vi "Pop Up Button Animator.vi"(5 "Button Ref":refnum<vi>, 7 "Msg Settings":T1={"Grow Time"=0.3, "Msg Time"=0.5, "Shrink Time"=0.1, "Msg Pos"={"Left"=170, "Top"=300}, "Button Size"={"Width"=169, "Height"=93}}, 8 "error in (no error)":errorcluster) -> (0 "error out":errorcluster)   [LabVIEW 2013]
uses:
  Message States.ctl
  <vilib>/Utility/miscctls.llb/LVBoundsTypeDef.ctl
panel:
  out "Message":string
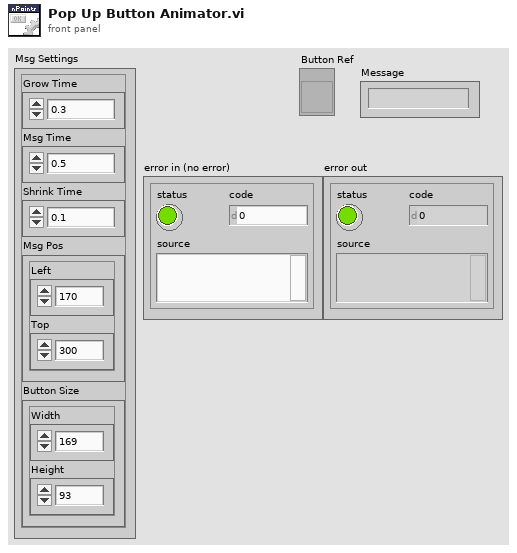
[diagram p1: front panel]
types:
  T1 = cluster{"Grow Time":dbl, "Msg Time":dbl, "Shrink Time":dbl, "Msg Pos":cluster{"Left":i32, "Top":i32}, "Button Size":cluster{"Width":i32, "Height":i32}}
  T2 = typedef "Message States.ctl" = enum16{"Reset", "PopUp", "Grow", "Message On", "Shrink", "Wait", "Quit"}
  T3 = typedef "LVBoundsTypeDef.ctl" = cluster{"Width":u32, "Height":u32}
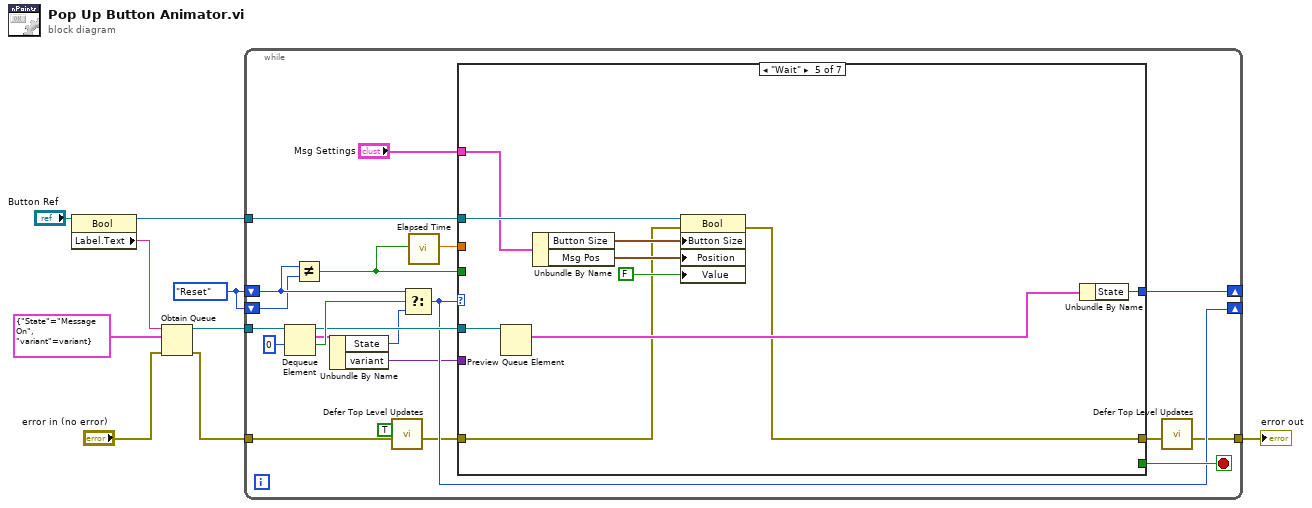
[diagram p0: block diagram]
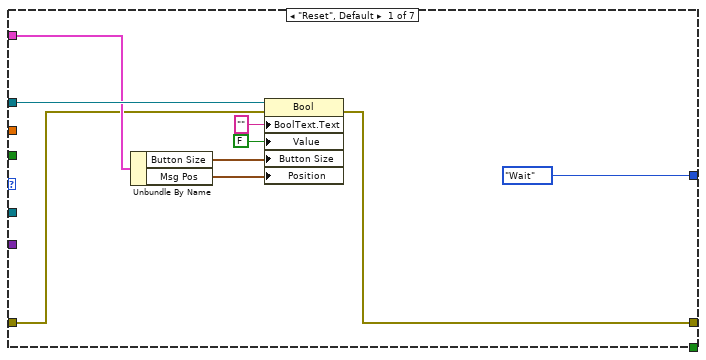
[diagram p2: hidden frame]
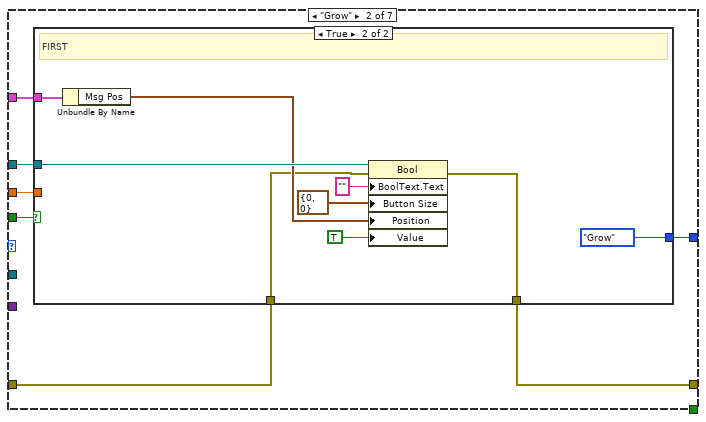
[diagram p3: hidden frame]
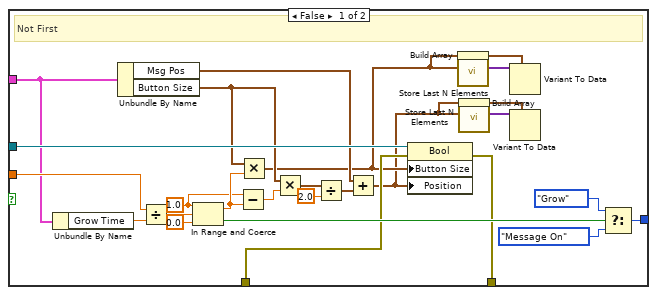
[diagram p4: hidden frame]
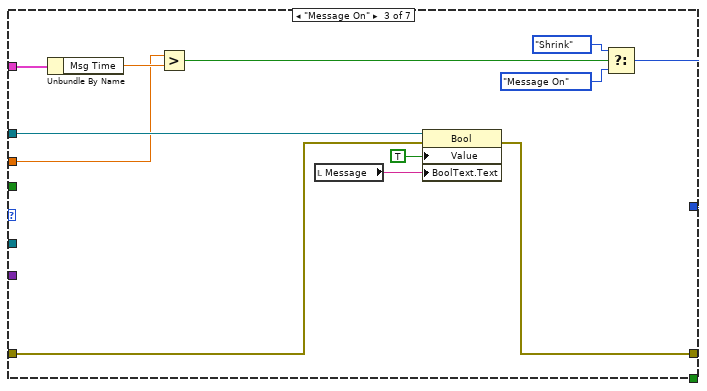
[diagram p5: hidden frame]
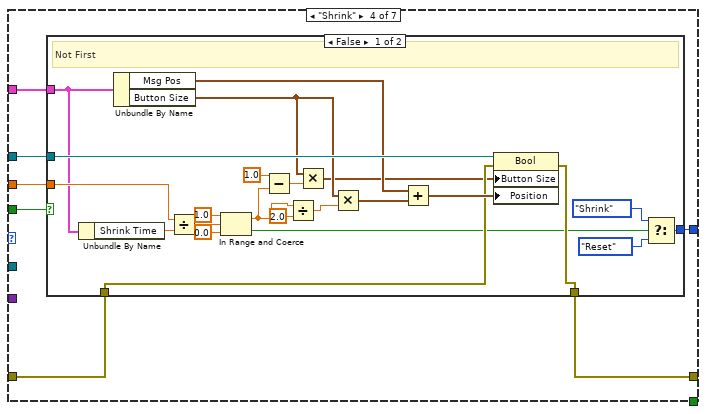
[diagram p6: hidden frame]
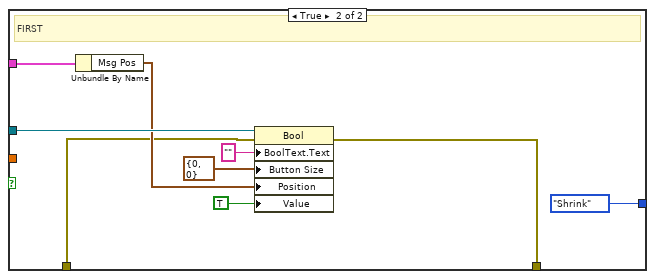
[diagram p7: hidden frame]
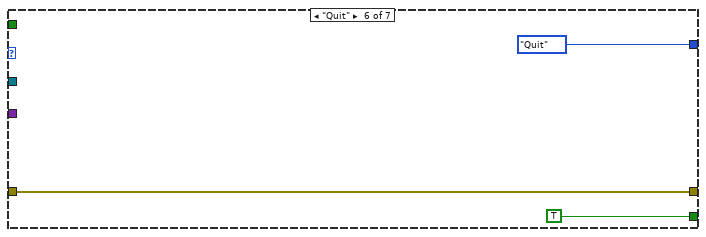
[diagram p8: hidden frame]
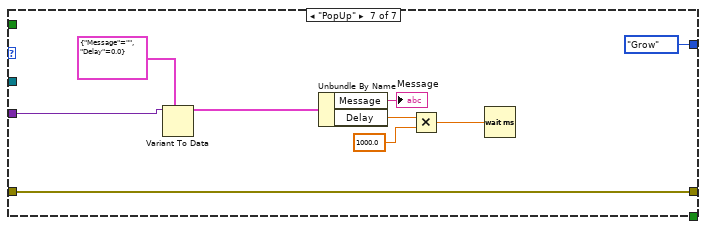
[diagram p9: hidden frame]
diagram:
  w8 = Message_States."Reset" ("Button State")
  n1 = property on="Property Node" class="Bool"(reference="Button Ref") -> (reference out=w2:refnum<vi>, "Label.Text"=w1:string)  [unwired: 1 in, 1 out]
  n2 = Obtain Queue(name (unnamed)=w1, element data type=cluster{"State":T2, "variant":variant} {"State"=enum."Message On", "variant"=variant}, error in (no error)="error in (no error)") -> (queue out=w9:refnum<queue>, error out=w5:errorcluster)  [unwired: 2 in, 1 out]
  n3 = while {
    tunnel: w9 -> [w30]
    tunnel: w2 -> [w27]
    shift-right: [w26] -> _
    shift-left: w8 -> [w22]
    shift-right: [w23] -> _
    shift-left: w8 -> [w21]
    tunnel: w5 -> [w13]
    tunnel: [w10] -> w4
    stop <- w28 stop-if-true
    n4 = Dequeue Element(queue=w30, timeout in ms (-1)=0) -> (queue out=w24:refnum<queue>, element=w16:cluster{"State":T2, "variant":variant}, timed out?=w25:bool)  [unwired: 1 in, 1 out]
    n5 = Not Equal?(x=w22, y=w21) -> (x != y?=w20:bool)
    n6 = Unbundle By Name(w16) -> ("State"=w17:T2, "variant"=w15:variant)
    n7 = call "Defer Top Level Updates.vi"("error in (no error)"=w13, "Defer Panel Updates (f)"=TRUE) -> ("error out"=w14:errorcluster)  [unwired: 5 in]
    n8 = Select(t=w22, s=w25, f=w17) -> (s? t:f=w23:T2)
    n9 = call "Elapsed Time"("Reset"=w20) -> ("Elapsed Time (s)"=w19:dbl)  [unwired: 11 in, 7 out]
    n10 = case shown="\"Wait\"" w23 {
      tunnel: [_ _ _ _ _ TRUE _] -> w28
      tunnel: w27 -> [w37 w46 w92 w98 w141 _ _]
      tunnel: [Message_States."Wait" ("Button State") w44 w85 w97 w135 Message_States."Quit" ("Button State") Message_States."Grow" ("Button State")] -> w26
      tunnel: w24 -> [_ _ _ _ w142 _ _]
      tunnel: w20 -> [_ w45 _ w96 _ _ _]
      tunnel: w19 -> [_ w43 w89 w99 _ _ _]
      tunnel: "Msg Settings" -> [w35 w42 w91 w100 w139 _ _]
      tunnel: w15 -> [_ _ _ _ _ _ w152]
      tunnel: [w31 w40 w83 w94 w133 w143 w154] -> w11
      tunnel: w14 -> [w32 w41 w84 w95 w134 w143 w154]
      frame "Reset", Default {
        n11 = Unbundle By Name(w35) -> ("Button Size"=w34:cluster{"Width":i32, "Height":i32}, "Msg Pos"=w33:cluster{"Left":i32, "Top":i32})
        n12 = property on="Property Node" class="Bool"(reference=w37, error in=w32, "BoolText.Text"="" ("Boolean Text.Text"), "Value"=FALSE, "Button Size"=w34, "Position"=w33) -> (error out=w31:errorcluster)  [unwired: 1 out]
      }
      frame "Grow" {
        n13 = case shown="True" w45 {
          tunnel: w46 -> [w70 w80]
          tunnel: [w67 Message_States."Grow" ("Button State")] -> w44
          tunnel: w43 -> [w63 _]
          tunnel: w42 -> [w61 w76]
          tunnel: w41 -> [w58 w74]
          tunnel: [w59 w73] -> w40
          frame False {
            w56 = 1.0 ("lower limit")
            # "Not First"
            n14 = Unbundle By Name(w61) -> ("Grow Time"=w62:dbl)
            n15 = Unbundle By Name(w61) -> ("Msg Pos"=w60:cluster{"Left":i32, "Top":i32}, "Button Size"=w53:cluster{"Width":i32, "Height":i32})
            n16 = Divide(x=w63, y=w62) -> (x/y=w72:dbl)
            n17 = In Range and Coerce(upper limit=w56, x=w72, lower limit=0.0) -> (coerced(x)=w57:dbl, In Range?=w66:bool)
            n18 = Subtract(x=w56, y=w57) -> (x-y=w55:dbl)
            n19 = Multiply(x=w53, y=w57) -> (x*y=w50:cluster{"Width":dbl, "Height":dbl})
            n20 = Multiply(x=w53, y=w55) -> (x*y=w54:cluster{"Width":dbl, "Height":dbl})
            n21 = Divide(x=w54, y=2.0 ("lower limit")) -> (x/y=w65:cluster{"Width":dbl, "Height":dbl})
            n22 = Add(x=w60, y=w65) -> (x+y=w48:cluster{dbl, dbl})
            n23 = property on="Property Node" class="Bool"(reference=w70, error in=w58, "Button Size"=w50, "Position"=w48) -> (error out=w59:errorcluster)  [unwired: 1 out]
            n24 = Build Array(w50) -> (w49:cluster{"Width":dbl, "Height":dbl}[])
            n25 = call <userlib>:"Store Last N Elements.vi"("Element"=w50) -> ("Element Array"=w52:variant[])  [unwired: 10 in]
            n26 = Build Array(w48) -> (w47:cluster{dbl, dbl}[])
            n27 = call <userlib>:"Store Last N Elements.vi"("Element"=w48) -> ("Element Array"=w51:variant[])  [unwired: 10 in]
            n28 = Variant To Data(type=w49, Variant=w52) -> ()  [unwired: 1 in, 2 out]
            n29 = Variant To Data(type=w47, Variant=w51) -> ()  [unwired: 1 in, 2 out]
            n30 = Select(t=Message_States."Grow" ("Button State"), s=w66, f=Message_States."Message On" ("Button State")) -> (s? t:f=w67:T2)
          }
          frame True {
            # "FIRST"
            n31 = Unbundle By Name(w76) -> ("Msg Pos"=w75:cluster{"Left":i32, "Top":i32})
            n32 = property on="Property Node" class="Bool"(reference=w80, error in=w74, "BoolText.Text"="" ("Boolean Text.Text"), "Button Size"=T3 {"Width"=0, "Height"=0}, "Position"=w75, "Value"=TRUE) -> (error out=w73:errorcluster)  [unwired: 1 out]
          }
        }
      }
      frame "Message On" {
        n33 = Unbundle By Name(w91) -> ("Msg Time"=w90:dbl)
        n34 = Greater?(x=w89, y=w90) -> (0:w88:bool)
        n35 = local read "Message"() -> (w82:string)
        n36 = property on="Property Node" class="Bool"(reference=w92, error in=w84, "Value"=TRUE, "BoolText.Text"=w82) -> (error out=w83:errorcluster)  [unwired: 1 out]
        n37 = Select(t=Message_States."Shrink" ("Button State"), s=w88, f=Message_States."Message On" ("Button State")) -> (s? t:f=w85:T2)
      }
      frame "Shrink" {
        n38 = case shown="False" w96 {
          tunnel: w98 -> [w120 w132]
          tunnel: [w117 Message_States."Shrink" ("Button State")] -> w97
          tunnel: w99 -> [w114 _]
          tunnel: w100 -> [w110 w127]
          tunnel: w95 -> [w108 w125]
          tunnel: [w107 w124] -> w94
          frame False {
            # "Not First"
            n39 = Unbundle By Name(w110) -> ("Shrink Time"=w113:dbl)
            n40 = Unbundle By Name(w110) -> ("Msg Pos"=w109:cluster{"Left":i32, "Top":i32}, "Button Size"=w104:cluster{"Width":i32, "Height":i32})
            n41 = Divide(x=w114, y=w113) -> (x/y=w123:dbl)
            n42 = In Range and Coerce(upper limit=1.0 ("lower limit"), x=w123, lower limit=0.0) -> (coerced(x)=w106:dbl, In Range?=w102:bool)
            n43 = Subtract(x=1.0 ("lower limit"), y=w106) -> (x-y=w111:dbl)
            n44 = Divide(x=w106, y=2.0 ("lower limit")) -> (x/y=w105:dbl)
            n45 = Multiply(x=w104, y=w111) -> (x*y=w101:cluster{"Width":dbl, "Height":dbl})
            n46 = Multiply(x=w104, y=w105) -> (x*y=w103:cluster{"Width":dbl, "Height":dbl})
            n47 = Add(x=w109, y=w103) -> (x+y=w115:cluster{dbl, dbl})
            n48 = property on="Property Node" class="Bool"(reference=w120, error in=w108, "Button Size"=w101, "Position"=w115) -> (error out=w107:errorcluster)  [unwired: 1 out]
            n49 = Select(t=Message_States."Shrink" ("Button State"), s=w102, f=Message_States."Reset" ("Button State")) -> (s? t:f=w117:T2)
          }
          frame True {
            # "FIRST"
            n50 = Unbundle By Name(w127) -> ("Msg Pos"=w126:cluster{"Left":i32, "Top":i32})
            n51 = property on="Property Node" class="Bool"(reference=w132, error in=w125, "BoolText.Text"="" ("Boolean Text.Text"), "Button Size"=T3 {"Width"=0, "Height"=0}, "Position"=w126, "Value"=TRUE) -> (error out=w124:errorcluster)  [unwired: 1 out]
          }
        }
      }
      frame "Wait" {
        n52 = Preview Queue Element(queue=w142) -> (element=w136:cluster{"State":T2, "variant":variant})  [unwired: 2 in, 3 out]
        n53 = Unbundle By Name(w139) -> ("Button Size"=w138:cluster{"Width":i32, "Height":i32}, "Msg Pos"=w137:cluster{"Left":i32, "Top":i32})
        n54 = property on="Property Node" class="Bool"(reference=w141, error in=w134, "Button Size"=w138, "Position"=w137, "Value"=FALSE) -> (error out=w133:errorcluster)  [unwired: 1 out]
        n55 = Unbundle By Name(w136) -> ("State"=w135:T2)
      }
      frame "Quit" {
      }
      frame "PopUp" {
        n56 = Variant To Data(type=cluster{"Message":string, "Delay":dbl} {"Message"="", "Delay"=0.0}, Variant=w152) -> (data=w151:cluster{"Message":string, "Delay":dbl})  [unwired: 1 in, 1 out]
        n57 = Unbundle By Name(w151) -> ("Message"=→"Message":string, "Delay"=w148:dbl)
        n58 = Multiply(x=w148, y=1000.0) -> (x*y=w146:dbl)
        n59 = Wait (ms)(milliseconds to wait=w146) -> ()  [unwired: 1 out]
      }
    }
    n60 = call "Defer Top Level Updates.vi"("error in (no error)"=w11) -> ("error out"=w10:errorcluster)  [unwired: 6 in]
  }
  "error out" <- w4
